vi "Connect.vi"(8 "error in":errorcluster) -> (0 "error out":errorcluster, 3 "CanHandleOut":T1)   [LabVIEW 2011, in "Konvolucio MCAN120803.lvlib"]
doc: "Connect the adapter."
uses:
  <instrlib>/Konvolucio MCAN120803/Konvolucio MCAN120803.lvlib
  <instrlib>/Konvolucio MCAN120803/Types/CanHandleType.ctl
  C:/Program Files/National Instruments/LabVIEW 2011/instr.lib/Konvolucio MCAN120803/Private/Konvolucio.MCAN120803.API.dll
  Private/Konvolucio.MCAN120803.API.dll
  <instrlib>/Konvolucio MCAN120803/Types/StateType.ctl
  <instrlib>/Konvolucio MCAN120803/Public/Attributes/AttrGetState.vi
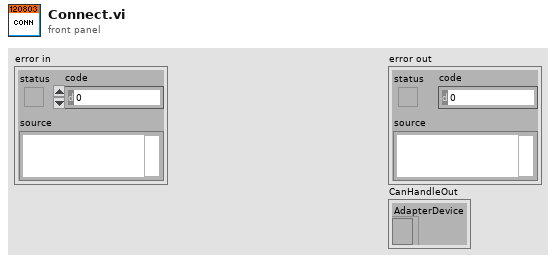
[diagram p1: front panel]
types:
  T1 = typedef "Konvolucio MCAN120803.lvlib/CanHandleType.ctl" = cluster{"AdapterDevice":refnum<k24>}
  T2 = typedef "Konvolucio MCAN120803.lvlib/StateType.ctl" = enum16{"SDEV_NONE", "SDEV_START", "SDEV_STOP", "SDEV_RESET", "SDEV_FAIL", "SDEV_IDLE"}
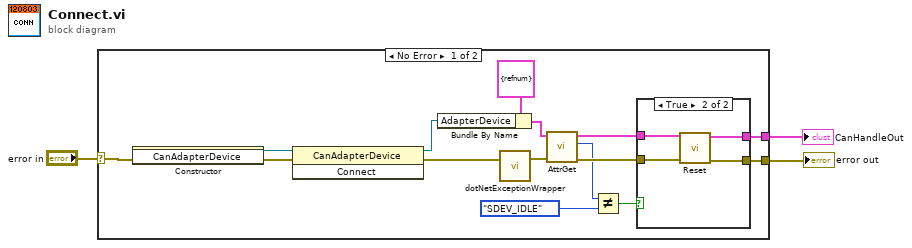
[diagram p0: block diagram]
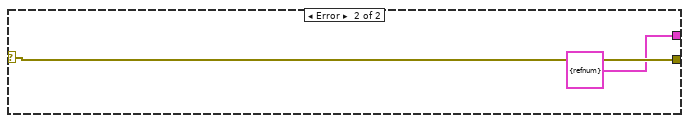
[diagram p3: hidden frame]
diagram:
  n1 = case shown="No Error" "error in" {
    selector: "error in" -> [w7 w26]
    tunnel: [w5 w26] -> w2
    tunnel: [w4 T1 {"AdapterDevice"=refnum} ("HandleOut")] -> w1
    frame No Error {
      n2 = constructor class="CanAdapterDevice"(error in=w7) -> (reference out=w8:refnum<k24>, error out=w9:errorcluster)  [unwired: 2 in, 1 out]
      n3 = invoke class="CanAdapterDevice" method="Connect"(reference=w8, error in=w9) -> (reference out=w11:refnum<k24>, error out=w6:errorcluster)  [unwired: 1 in, 1 out]
      n4 = Bundle By Name(cluster=T1 {"AdapterDevice"=refnum}, "AdapterDevice"=w11) -> (w12:T1)
      n5 = call <instrlib>:"dotNetExceptionWrapper.vi"("error in"=w6) -> ("error out"=w18:errorcluster)  [unwired: 2 in]
      n6 = call-poly <instrlib>:"AttrGet.vi"("error in"=w18, "CanHandleIn"=w12) -> ("error out"=w16:errorcluster, "State"=w14:T2, "CanHandleOut"=w17:T1)  [unwired: 7 in]
      n7 = Not Equal?(x=w14, y=StateType."SDEV_IDLE") -> (x != y?=w15:bool)
      n8 = case shown="True" w15 {
        tunnel: w16 -> [w19 w24]
        tunnel: w17 -> [w20 w23]
        tunnel: [w20 w22] -> w4
        tunnel: [w19 w21] -> w5
        frame False {
        }
        frame True {
          n9 = call <instrlib>:"Reset.vi"("error in"=w24, "CanHandleIn"=w23) -> ("error out"=w21:errorcluster, "CanHandleOut"=w22:T1)  [unwired: 8 in]
        }
      }
    }
    frame Error {
    }
  }
  "error out" <- w2
  "CanHandleOut" <- w1
